vi "Mod5DIOaus_ECD.vi"   [LabVIEW 2017]
uses:
  <vilib>/rvi/eio/common/nirviEmuTemplateMethod_errors.vi
  <vilib>/eio/EIONode/EIONode.xnode
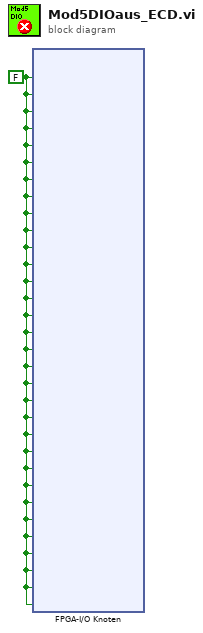
[diagram p0: block diagram]
diagram:
  w1 = FALSE ("Mod5/DIO0")
  n1 = xnode "FPGA-I/O Knoten"("Mod5/DIO0"=w1, "Mod5/DIO1"=w1, "Mod5/DIO2"=w1, "Mod5/DIO3"=w1, "Mod5/DIO4"=w1, "Mod5/DIO5"=w1, "Mod5/DIO6"=w1, "Mod5/DIO7"=w1, "Mod5/DIO8"=w1, "Mod5/DIO9"=w1, "Mod5/DIO10"=w1, "Mod5/DIO11"=w1, "Mod5/DIO12"=w1, "Mod5/DIO13"=w1, "Mod5/DIO14"=w1, "Mod5/DIO15"=w1, "Mod5/DIO16"=w1, "Mod5/DIO17"=w1, "Mod5/DIO18"=w1, "Mod5/DIO19"=w1, "Mod5/DIO20"=w1, "Mod5/DIO21"=w1, "Mod5/DIO22"=w1, "Mod5/DIO23"=w1, "Mod5/DIO24"=w1, "Mod5/DIO25"=w1, "Mod5/DIO26"=w1, "Mod5/DIO27"=w1, "Mod5/DIO28"=w1, "Mod5/DIO29"=w1, "Mod5/DIO30"=w1, "Mod5/DIO31"=w1) -> ()  [unwired: 32 in, 32 out]
